vi "Get Library.vi"(8 "error in":errorcluster, 10 "library name":string, 11 "project ref":refnum<vi>) -> (0 "error out":errorcluster, 1 "found":bool, 2 "library item":refnum<vi>, 3 "project ref out":refnum<vi>)   [LabVIEW 2021, in "InstrumentStudio Plug-In Editor.lvlib"]
uses:
  InstrumentStudio Plug-In Editor.lvlib
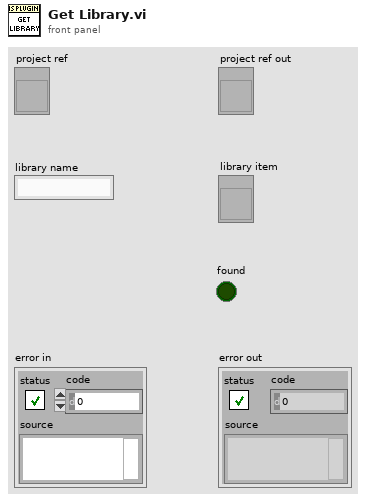
[diagram p1: front panel]
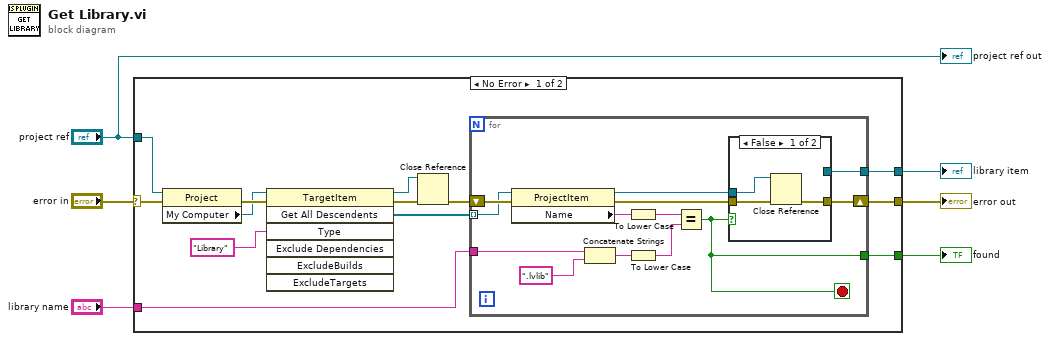
[diagram p0: block diagram]
diagram:
  n1 = case shown="No Error" "error in" {
    selector: "error in" -> [w17 w38]
    tunnel: "project ref" -> [w12 _]
    tunnel: [w16 w38] -> w4
    tunnel: "library name" -> [w10 _]
    tunnel: [w9 _] -> w2
    tunnel: [w8 _] -> w1
    frame No Error {
      n2 = property class="Project"(reference=w12, error in=w17) -> (error out=w19:errorcluster, "My Computer"=w11:refnum<vi>)  [unwired: 1 out]
      n3 = invoke class="TargetItem" method="Get All Descendents"(reference=w11, error in=w19, "Type"="Library") -> (reference out=w13:refnum<vi>, error out=w15:errorcluster, "All Descendents"=w18:refnum<vi>[])  [unwired: 4 in, 4 out]
      n4 = Close Reference(reference=w13, error in (no error)=w15) -> (error out=w14:errorcluster)
      n5 = for {
        tunnel: w18 -> [w31] mode=indexing
        shift-right: [w29] -> w16
        shift-left: w14 -> [w32]
        tunnel: w10 -> [w27]
        tunnel: [w21] -> w9
        tunnel: [w20] -> w8
        stop <- w20 stop-if-true
        n6 = property class="ProjectItem"(reference=w31, error in=w32) -> (reference out=w28:refnum<vi>, error out=w30:errorcluster, "Name"=w23:string)
        n7 = Concatenate Strings(w27, ".lvlib" ("string")) -> (w25:string)
        n8 = To Lower Case(string=w23) -> (all lower case string=w22:string)
        n9 = To Lower Case(string=w25) -> (all lower case string=w24:string)
        n10 = Equal?(x=w22, y=w24) -> (x = y?=w20:bool)
        n11 = case shown="False" w20 {
          tunnel: [w34 w37] -> w29
          tunnel: w30 -> [w35 w37]
          tunnel: w28 -> [w33 w36]
          tunnel: [_ w36] -> w21
          frame False {
            n12 = Close Reference(reference=w33, error in (no error)=w35) -> (error out=w34:errorcluster)
          }
          frame True {
          }
        }
      }
    }
    frame Error {
    }
  }
  "error out" <- w4
  "library item" <- w2
  "found" <- w1
  "project ref out" <- "project ref"
